vi "UMLEditor NewPrintDialog.vi"(5 "error in (no error)":errorcluster={"status"=FALSE, "code"=200021, "source"="DAQmx Write (Analog DBL 1Chan 1Samp).vi"}) -> (15 "PrinterInfo":T1={"PrinterName"="\\\\PLUTO\\Canon GP225", "Copies"=1, "PrintToFile"=FALSE, "orientation"=0, "PaperSize"=1} {"PaperSize" items=["PaperLetter"=1, "PaperLetterSmall"=2, "PaperTabloid"=3, "PaperLedger"=4, "PaperLegal"=5, "PaperStatement"=6, "PaperExecutive"=7, "PaperA3"=8, "PaperA4"=9, "PaperA4Small"=10, "PaperA5"=11, "PaperB4"=12, "PaperB5"=13, "PaperFolio"=14, "PaperQuarto"=15, "Paper10x14"=16, "Paper11x17"=17, "PaperNote"=18, "PaperEnvelop9"=19, "PaperEnvelop10"=20, "PaperEnvelop11"=21, "PaperEnvelop12"=22, "PaperEnvelop14"=23, "PaperCSheet"=24, "PaperDSheet"=25, "PaperESheet"=26, "PaperEnvelopDL"=27, "PaperEnvelopC5"=28, "PaperEnvelopC3"=29, "PaperEnvelopC4"=30, "PaperEnvelopC6"=31, "PaperEnvelopC65"=32, "PaperEnvelopB4"=33, "PaperEnvelopB5"=34, "PaperEnvelopB6"=35, "PaperEnvelopItaly"=36, "PaperEnvelopMonarch"=37, "PaperEnvelopPersonal"=38, "PaperFanFoldUS"=39, "PaperFanFoldStandardGerman"=40, "PaperFanFoldLegalGerman"=41, "PaperISOB4"=42, "PaperJapanesePostcard"=43, "Paper9X11"=44, "Paper10X11"=45, "Paper15X11"=46, "PaperEnvelopInvite"=47, "PaperLetterExtra"=50, "PaperLegalExtra"=51, "PaperTabloidExtra"=52, "PaperA4Extra"=53, "PaperLetterTransverse"=54, "PaperA4Transverse"=55, "PaperLetterExtraTransverse"=56, "PaperAPlus"=57, "PaperBPlus"=58, "PaperLetterPlus"=59, "PaperA4Plus"=60, "PaperA5Transverse"=61, "PaperB5Transverse"=62, "PaperA3Extra"=63, "PaperA5Extra"=64, "PaperB5Extra"=65, "PaperA2"=66, "PaperA3Transverse"=67, "PaperA3ExtraTransverse"=68]; "orientation" items=["portrait", "landscape"]}, 16 "Cancelled":bool, 19 "error out":errorcluster={"status"=FALSE, "code"=200021, "source"="DAQmx Write (Analog DBL 1Chan 1Samp).vi"})   [LabVIEW 2020]
uses:
  <resource>/Framework/Providers/Open_GDS/UML/UMLEditor/UMLEditor PrinterSettings.ctl
  Instance           1 32Saved   UMLEditor NewPrintDialog .vi
  <vilib>/Utility/NIReport.llb/NI_ReportGenerationCore.lvlib
panel:
  in  "Paper Size:":i32(ring)=1 items=["PaperLetter"=1, "PaperLetterSmall"=2, "PaperTabloid"=3, "PaperLedger"=4, "PaperLegal"=5, "PaperStatement"=6, "PaperExecutive"=7, "PaperA3"=8, "PaperA4"=9, "PaperA4Small"=10, "PaperA5"=11, "PaperB4"=12, "PaperB5"=13, "PaperFolio"=14, "PaperQuarto"=15, "Paper10x14"=16, "Paper11x17"=17, "PaperNote"=18, "PaperEnvelop9"=19, "PaperEnvelop10"=20, "PaperEnvelop11"=21, "PaperEnvelop12"=22, "PaperEnvelop14"=23, "PaperCSheet"=24, "PaperDSheet"=25, "PaperESheet"=26, "PaperEnvelopDL"=27, "PaperEnvelopC5"=28, "PaperEnvelopC3"=29, "PaperEnvelopC4"=30, "PaperEnvelopC6"=31, "PaperEnvelopC65"=32, "PaperEnvelopB4"=33, "PaperEnvelopB5"=34, "PaperEnvelopB6"=35, "PaperEnvelopItaly"=36, "PaperEnvelopMonarch"=37, "PaperEnvelopPersonal"=38, "PaperFanFoldUS"=39, "PaperFanFoldStandardGerman"=40, "PaperFanFoldLegalGerman"=41, "PaperISOB4"=42, "PaperJapanesePostcard"=43, "Paper9X11"=44, "Paper10X11"=45, "Paper15X11"=46, "PaperEnvelopInvite"=47, "PaperLetterExtra"=50, "PaperLegalExtra"=51, "PaperTabloidExtra"=52, "PaperA4Extra"=53, "PaperLetterTransverse"=54, "PaperA4Transverse"=55, "PaperLetterExtraTransverse"=56, "PaperAPlus"=57, "PaperBPlus"=58, "PaperLetterPlus"=59, "PaperA4Plus"=60, "PaperA5Transverse"=61, "PaperB5Transverse"=62, "PaperA3Extra"=63, "PaperA5Extra"=64, "PaperB5Extra"=65, "PaperA2"=66, "PaperA3Transverse"=67, "PaperA3ExtraTransverse"=68]
  in  "Name:":u16(ring) items=["Microsoft Office Document Image Writer", "Lexmark Z53 Color Jetprinter", "HP Business Inkjet 2200/2250 (HPA)", "Auto DeskJet 990cxi on PLUTO", "Auto Canon GP225 on PLUTO", "\\\\PLUTO\\DeskJet 990cxi"]
  in  "Landscape":bool
  in  "Portrait":bool=TRUE
  in  "Number of copies:":i32=1 min=1
  in  "Cancel":bool
  in  "Ok":bool
  in  "Locals":T2
  # "Configure your printer"
  # "Select printer and configure the output"
  # "Printer"
  # "Name:"
  # "Paper Orientation"
  # "Copies"
  # "3"
  # "2"
  # "1"
  # "A"
  # "A"
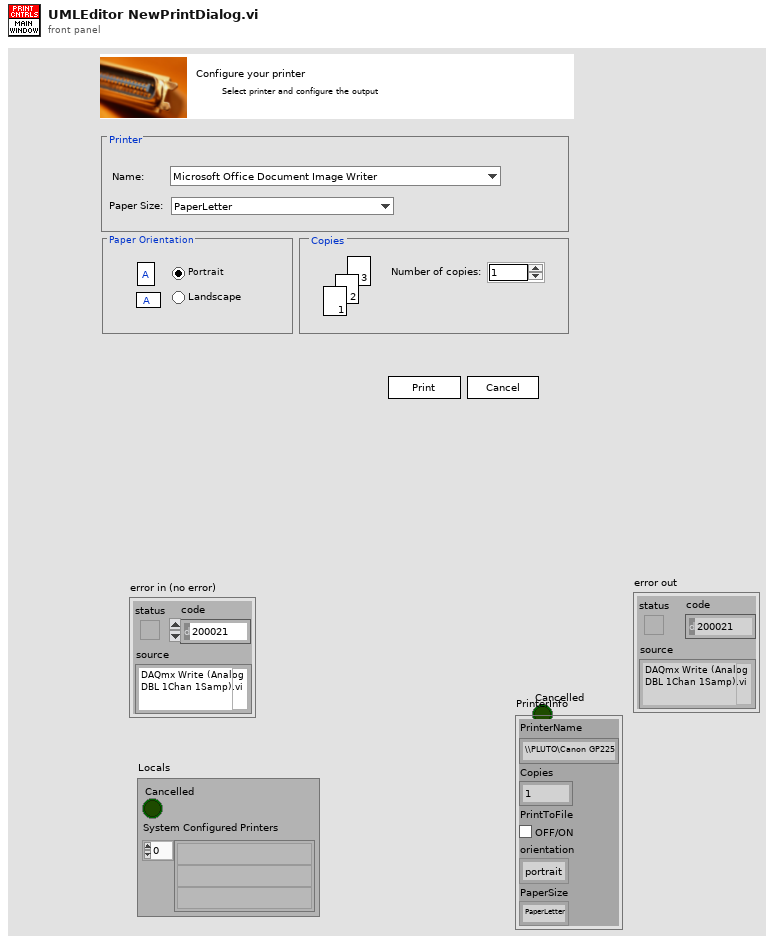
[diagram p1: front panel]
types:
  T1 = typedef "UMLEditor PrinterSettings.ctl" = cluster{"PrinterName":string, "Copies":i32, "PrintToFile":bool, "orientation":u16, "PaperSize":i32}
  T2 = cluster{"Cancelled":bool, "System Configured Printers":string[]}
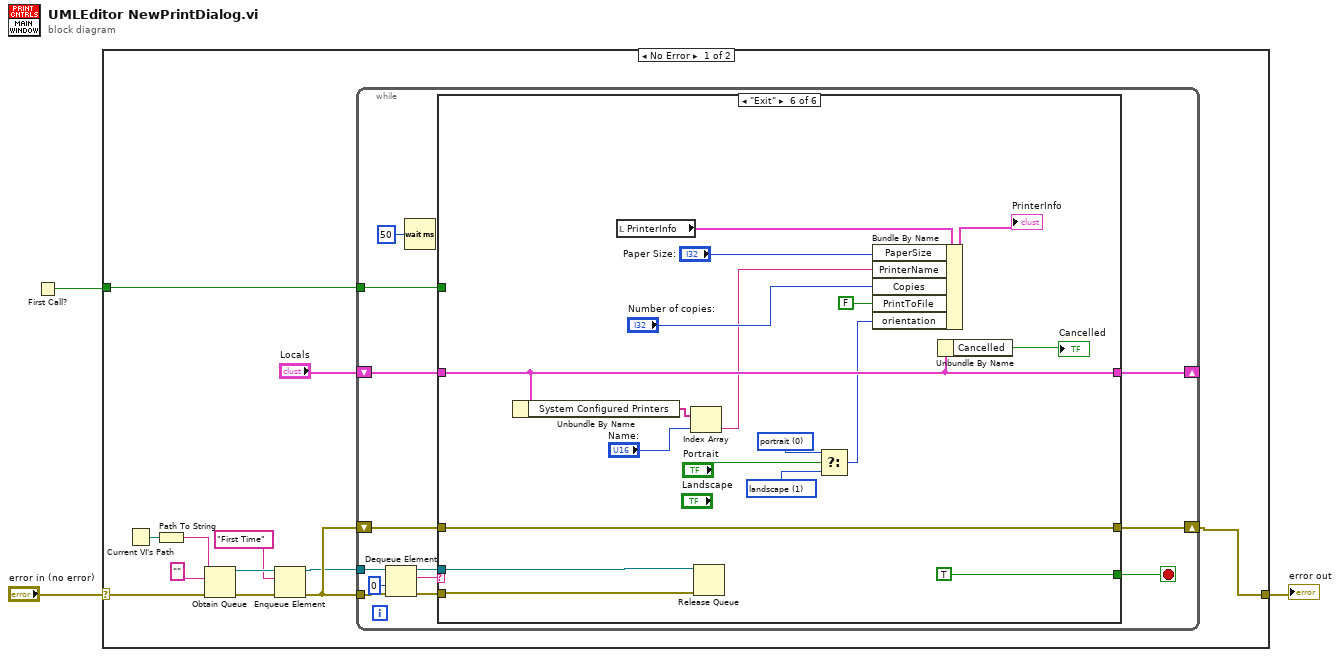
[diagram p0: block diagram]
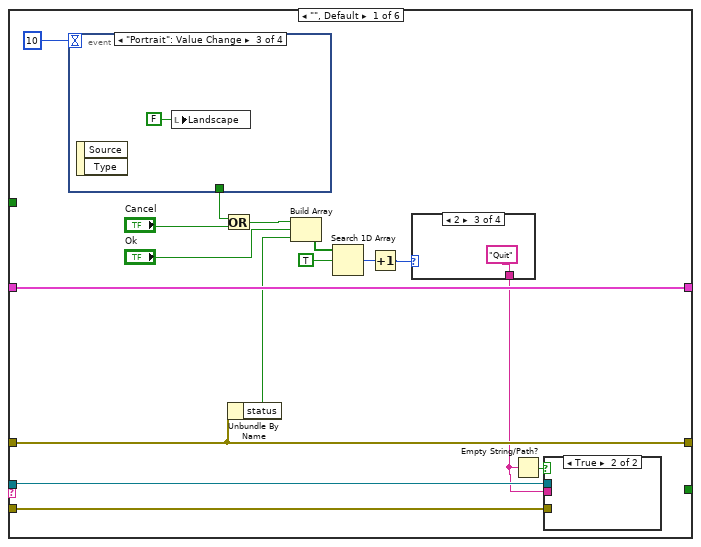
[diagram p2: hidden frame]
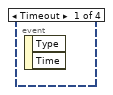
[diagram p3: hidden frame]
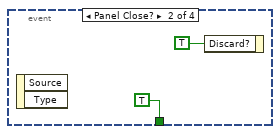
[diagram p4: hidden frame]
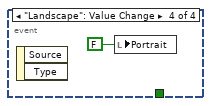
[diagram p5: hidden frame]
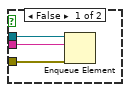
[diagram p6: hidden frame]
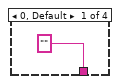
[diagram p7: hidden frame]
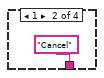
[diagram p8: hidden frame]
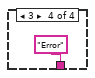
[diagram p9: hidden frame]
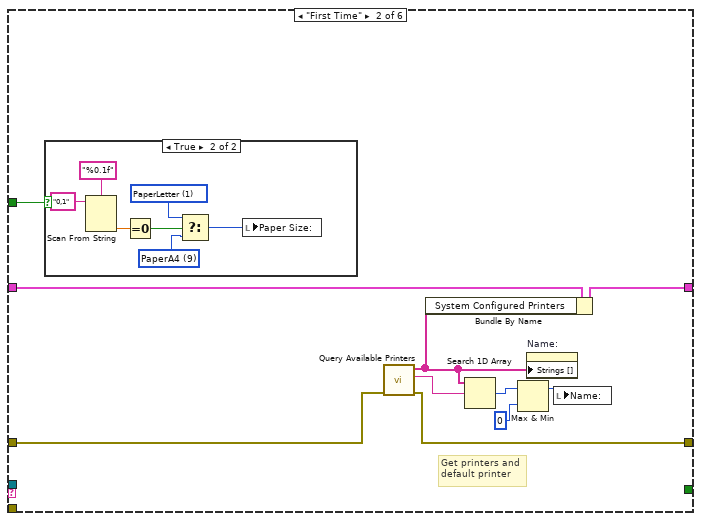
[diagram p10: hidden frame]
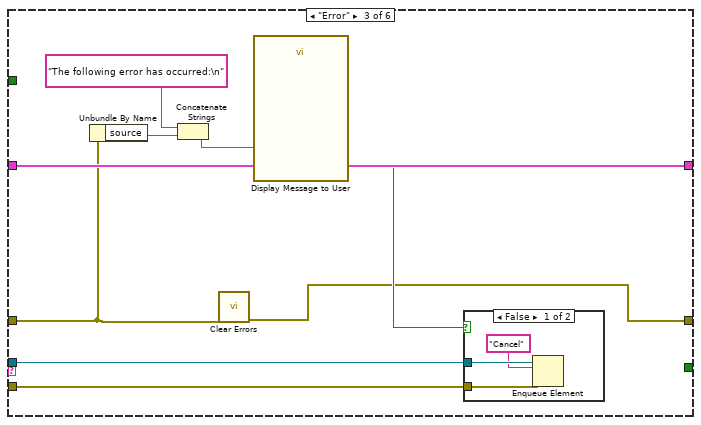
[diagram p12: hidden frame]
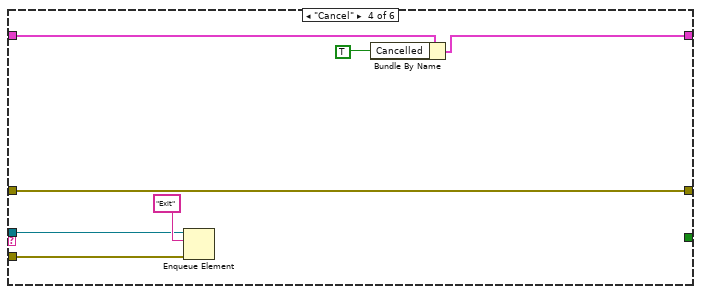
[diagram p14: hidden frame]
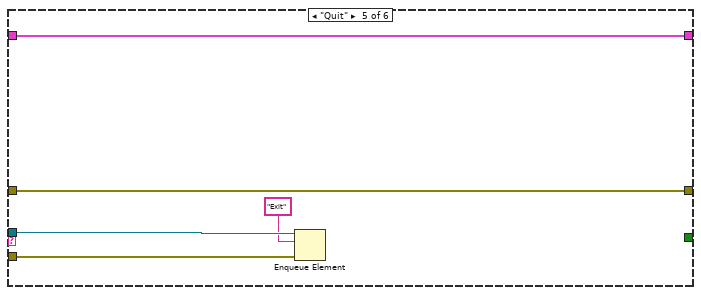
[diagram p15: hidden frame]
diagram:
  n1 = First Call?() -> (First Call?: T/F=w1:bool)
  n2 = case shown="No Error" "error in (no error)" {
    selector: "error in (no error)" -> [w15 w115]
    tunnel: [w6 w115] -> w2
    tunnel: w1 -> [w4 _]
    frame No Error {
      n3 = Current VI's Path() -> (path=w14:path)
      n4 = Path To String(path=w14) -> (string=w13:string)
      n5 = Obtain Queue(name (unnamed)=w13, element data type="", error in (no error)=w15) -> (queue out=w10:refnum<queue>, error out=w11:errorcluster)  [unwired: 2 in, 1 out]
      n6 = Enqueue Element(queue=w10, element="First Time", error in (no error)=w11) -> (queue out=w7:refnum<queue>, error out=w8:errorcluster)  [unwired: 2 out]
      n7 = while {
        shift-right: [w22] -> w6
        shift-left: w8 -> [w23]
        tunnel: w8 -> [w28]
        tunnel: w7 -> [w27]
        shift-right: [w19] -> _
        shift-left: "Locals" -> [w20]
        tunnel: w4 -> [w16]
        stop <- w21 stop-if-true
        n8 = Dequeue Element(queue=w27, timeout in ms (-1)=0, error in (no error)=w28) -> (queue out=w24:refnum<queue>, element=w25:string, error out=w26:errorcluster)  [unwired: 1 out]
        n9 = Wait (ms)(milliseconds to wait=u32 50) -> ()  [unwired: 1 out]
        n10 = case shown="\"Exit\"" w25 {
          tunnel: w26 -> [w38 _ w76 w89 w94 w111]
          tunnel: w24 -> [w37 _ w75 w88 w93 w112]
          tunnel: w23 -> [w43 w64 w74 w91 w95 w113]
          tunnel: [w43 w63 w73 w91 w95 w113] -> w22
          tunnel: [_ _ _ _ _ TRUE] -> w21
          tunnel: w20 -> [w44 w62 w81 w87 w96 w106]
          tunnel: [w44 w61 w81 w86 w96 w106] -> w19
          tunnel: w16 -> [_ w56 _ _ _ _]
          frame "", Default {
            n11 = event shown="[2] \"Portrait\": Value Change" {
              selector: _ -> [_ _ _ _]
              dyn-events: _ -> [_ _ _ _]
              timeout: 10 -> [_ _ _ _]
              tunnel: [_ TRUE ("Discard?") _ _] -> w32
              event Timeout {
                n12 = event-data() -> ()  [unwired: 3 out]
              }
              event Panel Close? {
                n13 = event-data() -> ()  [unwired: 3 out]
                n14 = event-data("Discard?"=TRUE) -> ()  [unwired: 1 in, 1 out]
              }
              event "Portrait": Value Change {
                n15 = event-data() -> ()  [unwired: 3 out]
                n16 = local write "Landscape"(FALSE ("Landscape")) -> ()
              }
              event "Landscape": Value Change {
                n17 = event-data() -> ()  [unwired: 3 out]
                n18 = local write "Portrait"(FALSE ("Portrait")) -> ()
              }
            }
            n19 = Or(x=w32, y="Cancel") -> (x .or. y?=w33:bool)
            n20 = Unbundle By Name(w43) -> ("status"=w29:bool)
            n21 = Build Array(w33, "Ok", w29) -> (w42:bool[])
            n22 = Search 1D Array(1D array=w42, element=TRUE) -> (index of element=w40:i32)  [unwired: 1 out]
            n23 = Increment(x=w40) -> (x+1=w39:i32)
            n24 = case shown="2" w39 {
              tunnel: ["" "Cancel" "Quit" "Error"] -> w35
              frame 0, Default {
              }
              frame 1 {
              }
              frame 2 {
              }
              frame 3 {
              }
            }
            n25 = Empty String/Path?(string/path=w35) -> (empty?=w36:bool)
            n26 = case shown="True" w36 {
              tunnel: w38 -> [w51 _]
              tunnel: w37 -> [w50 _]
              tunnel: w35 -> [w49 _]
              frame False {
                n27 = Enqueue Element(queue=w50, element=w49, error in (no error)=w51) -> ()  [unwired: 4 out]
              }
              frame True {
              }
            }
          }
          frame "First Time" {
            # "Get printers and\ndefault printer"
            n28 = case shown="True" w56 {
              frame False {
              }
              frame True {
                w67 = 9 items=["PaperLetter"=1, "PaperLetterSmall"=2, "PaperTabloid"=3, "PaperLedger"=4, "PaperLegal"=5, "PaperStatement"=6, "PaperExecutive"=7, "PaperA3"=8, "PaperA4"=9, "PaperA4Small"=10, "PaperA5"=11, "PaperB4"=12, "PaperB5"=13, "PaperFolio"=14, "PaperQuarto"=15, "Paper10x14"=16, "Paper11x17"=17, "PaperNote"=18, "PaperEnvelop9"=19, "PaperEnvelop10"=20, "PaperEnvelop11"=21, "PaperEnvelop12"=22, "PaperEnvelop14"=23, "PaperCSheet"=24, "PaperDSheet"=25, "PaperESheet"=26, "PaperEnvelopDL"=27, "PaperEnvelopC5"=28, "PaperEnvelopC3"=29, "PaperEnvelopC4"=30, "PaperEnvelopC6"=31, "PaperEnvelopC65"=32, "PaperEnvelopB4"=33, "PaperEnvelopB5"=34, "PaperEnvelopB6"=35, "PaperEnvelopItaly"=36, "PaperEnvelopMonarch"=37, "PaperEnvelopPersonal"=38, "PaperFanFoldUS"=39, "PaperFanFoldStandardGerman"=40, "PaperFanFoldLegalGerman"=41, "PaperISOB4"=42, "PaperJapanesePostcard"=43, "Paper9X11"=44, "Paper10X11"=45, "Paper15X11"=46, "PaperEnvelopInvite"=47, "PaperLetterExtra"=50, "PaperLegalExtra"=51, "PaperTabloidExtra"=52, "PaperA4Extra"=53, "PaperLetterTransverse"=54, "PaperA4Transverse"=55, "PaperLetterExtraTransverse"=56, "PaperAPlus"=57, "PaperBPlus"=58, "PaperLetterPlus"=59, "PaperA4Plus"=60, "PaperA5Transverse"=61, "PaperB5Transverse"=62, "PaperA3Extra"=63, "PaperA5Extra"=64, "PaperB5Extra"=65, "PaperA2"=66, "PaperA3Transverse"=67, "PaperA3ExtraTransverse"=68] ("Paper Size")
                w68 = 1 items=["PaperLetter"=1, "PaperLetterSmall"=2, "PaperTabloid"=3, "PaperLedger"=4, "PaperLegal"=5, "PaperStatement"=6, "PaperExecutive"=7, "PaperA3"=8, "PaperA4"=9, "PaperA4Small"=10, "PaperA5"=11, "PaperB4"=12, "PaperB5"=13, "PaperFolio"=14, "PaperQuarto"=15, "Paper10x14"=16, "Paper11x17"=17, "PaperNote"=18, "PaperEnvelop9"=19, "PaperEnvelop10"=20, "PaperEnvelop11"=21, "PaperEnvelop12"=22, "PaperEnvelop14"=23, "PaperCSheet"=24, "PaperDSheet"=25, "PaperESheet"=26, "PaperEnvelopDL"=27, "PaperEnvelopC5"=28, "PaperEnvelopC3"=29, "PaperEnvelopC4"=30, "PaperEnvelopC6"=31, "PaperEnvelopC65"=32, "PaperEnvelopB4"=33, "PaperEnvelopB5"=34, "PaperEnvelopB6"=35, "PaperEnvelopItaly"=36, "PaperEnvelopMonarch"=37, "PaperEnvelopPersonal"=38, "PaperFanFoldUS"=39, "PaperFanFoldStandardGerman"=40, "PaperFanFoldLegalGerman"=41, "PaperISOB4"=42, "PaperJapanesePostcard"=43, "Paper9X11"=44, "Paper10X11"=45, "Paper15X11"=46, "PaperEnvelopInvite"=47, "PaperLetterExtra"=50, "PaperLegalExtra"=51, "PaperTabloidExtra"=52, "PaperA4Extra"=53, "PaperLetterTransverse"=54, "PaperA4Transverse"=55, "PaperLetterExtraTransverse"=56, "PaperAPlus"=57, "PaperBPlus"=58, "PaperLetterPlus"=59, "PaperA4Plus"=60, "PaperA5Transverse"=61, "PaperB5Transverse"=62, "PaperA3Extra"=63, "PaperA5Extra"=64, "PaperB5Extra"=65, "PaperA2"=66, "PaperA3Transverse"=67, "PaperA3ExtraTransverse"=68] ("Paper Size")
                n29 = Scan From String(format string="%0.1f", input string="0,1") -> (output 1=w70:dbl)  [unwired: 2 in, 4 out]
                n30 = Equal To 0?(x=w70) -> (x = 0?=w69:bool)
                n31 = Select(t=w68, s=w69, f=w67) -> (s? t:f=w66:i32)
                n32 = local write "Paper Size:"(w66) -> ()
              }
            }
            n33 = call <vilib>:"Query Available Printers.vi"("error in (no error)"=w64) -> ("error out"=w63:errorcluster, "default printer"=w65:string, "system configured printers"=w60:string[])  [unwired: 8 out]
            n34 = Bundle By Name(cluster=w62, "System Configured Printers"=w60) -> (w61:T2)
            n35 = Search 1D Array(1D array=w60, element=w65) -> (index of element=w59:i32)  [unwired: 1 out]
            n36 = Max & Min(x=w59, y=0) -> (max(x,y)=w57:i32)  [unwired: 1 out]
            n37 = property on="Name:" class="Ring (strict)"("Strings []"=w60) -> ()  [unwired: 2 in, 2 out]
            n38 = local write "Name:"(w57) -> ()
          }
          frame "Error" {
            n39 = Unbundle By Name(w74) -> ("source"=w79:string)
            n40 = Concatenate Strings("The following error has occurred:\n" ("string"), w79) -> (w78:string)
            n41 = call <vilib>:"Clear Errors.vi"("error in (no error)"=w74) -> ("error out"=w73:errorcluster)  [unwired: 1 in, 5 out]
            n42 = call "Display Message to User"("Message"=w78) -> ("Ignore"=w77:bool)  [unwired: 2 in, 8 out]
            n43 = case shown="False" w77 {
              tunnel: w76 -> [w83 _]
              tunnel: w75 -> [w84 _]
              frame False {
                n44 = Enqueue Element(queue=w84, element="Cancel", error in (no error)=w83) -> ()  [unwired: 4 out]
              }
              frame True {
              }
            }
          }
          frame "Cancel" {
            n45 = Enqueue Element(queue=w88, element="Exit", error in (no error)=w89) -> ()  [unwired: 4 out]
            n46 = Bundle By Name(cluster=w87, "Cancelled"=TRUE) -> (w86:T2)
          }
          frame "Quit" {
            n47 = Enqueue Element(queue=w93, element="Exit", error in (no error)=w94) -> ()  [unwired: 4 out]
          }
          frame "Exit" {
            w99 = u16 1 items=["portrait", "landscape"] ("orientation (portrait)")
            w100 = u16 0 items=["portrait", "landscape"] ("orientation (portrait)")
            n48 = Unbundle By Name(w106) -> ("System Configured Printers"=w105:string[])
            n49 = local read "PrinterInfo"() -> (w110:T1)
            n50 = Index Array(array=w105, index="Name:") -> (element=w103:string)
            n51 = Release Queue(queue=w112, error in (no error)=w111) -> ()  [unwired: 4 out]
            n52 = Select(t=w100, s="Portrait", f=w99) -> (s? t:f=w101:u16)
            n53 = Bundle By Name(cluster=w110, "PaperSize"="Paper Size:", "PrinterName"=w103, "Copies"="Number of copies:", "PrintToFile"=FALSE, "orientation"=w101) -> (→"PrinterInfo":T1)
            n54 = Unbundle By Name(w106) -> ("Cancelled"=→"Cancelled":bool)
          }
        }
      }
    }
    frame Error {
    }
  }
  "error out" <- w2
